vi "BuildMenu3.vi"(8 "Click Type":T1, 9 "Point":T2, 10 "XRef":refnum<vi>, 11 "State In":T10={"Input Type"=variant(dbl 0.0), "Width"=0, "Typedef Name"="", "Value Type"=variant, "Selection"=0, "Options"=[], "Selections"=[], "Display Selections"=[], "Element Names"=[], "Typedef Name Width"=0, "Display Selection Width"=[], "Code Generated"=FALSE, "Write Lock"=FALSE, "Is DVR"=FALSE}) -> (1 "Show Standard Items? (Popup click only)":bool=TRUE, 2 "Menu Specification":T4)   [LabVIEW 2015, in "Read-Write-Signals.xnode"]
doc: "This ability VI is used to describe the menu LabVIEW will display in response to a popup (right) click or a ShowMenu reply from OperateClick.\n \n Click Type is the type of click that led to this call of the ability. Point is the location of the user's popup click, and is relative to the top-left corner of your XNode's bounds. You may use this point to make your popup sensitive to the location that was clicked. Show Standard Items? is applicable only if Click Type is Popup, and tells LabVIEW whether it should include the standard popup items that are included on every node in LabVIEW.\n \n Menu Specification is an array of clusters describing the menu.\n Item: A string that will appear in the menu.\n Id: A string that identifies this item and will be passed to SelectMenu3.\n StartSub: The current string will be the header for a pull right menu.\n EndSub: The current string will be the last item in a pull right menu.\n Checked: The current item will have a check mark next to it.\n Disabled: The current item will be diabled and greyed out.\n Separator: The current item will be a separator. Item string is not displayed.\n Help: The text that should be displayed in context help when this menu item is hovered over. This functionality is currently not implemented.\n \n The index from this array will be an input to SelectMenu3.\n \n Remember to localize the strings in your menu.\n\nDefault behavior: Only show standard items for a popup click, show nothing for operate click.\n\nThis ability does not provide UI and OS messages are not handled.\n\nSee also: SelectMenu3"
uses:
  Read-Write-Signals.xnode
  State.ctl
  Read-Write-Signals Item.ctl
  Read-Write-Signals Sub Item.ctl
  Read-Write-Signals Sub Item Type.ctl
  Read-Write-Signals Selection.ctl
  Read-Write-Signals Display Selection.ctl
  <vilib>/XNodeSupport/XNodeMenuSpecs3.ctl
  <vilib>/XNodeSupport/XNodeMenuSpec3.ctl
  <vilib>/XNodeSupport/XNodeString.ctl
  <vilib>/XNodeSupport/XNodeBool.ctl
  <vilib>/XNodeSupport/XNodeStandardHelpInfo.ctl
  <vilib>/XNodeSupport/XNodePath.ctl
  <vilib>/XNodeSupport/XNodePoint.ctl
  <vilib>/XNodeSupport/XNodeInt.ctl
  <vilib>/XNodeSupport/XNodeClickTypes.ctl
  <vilib>/XNodeSupport/NI_XNodeSupport.lvlib
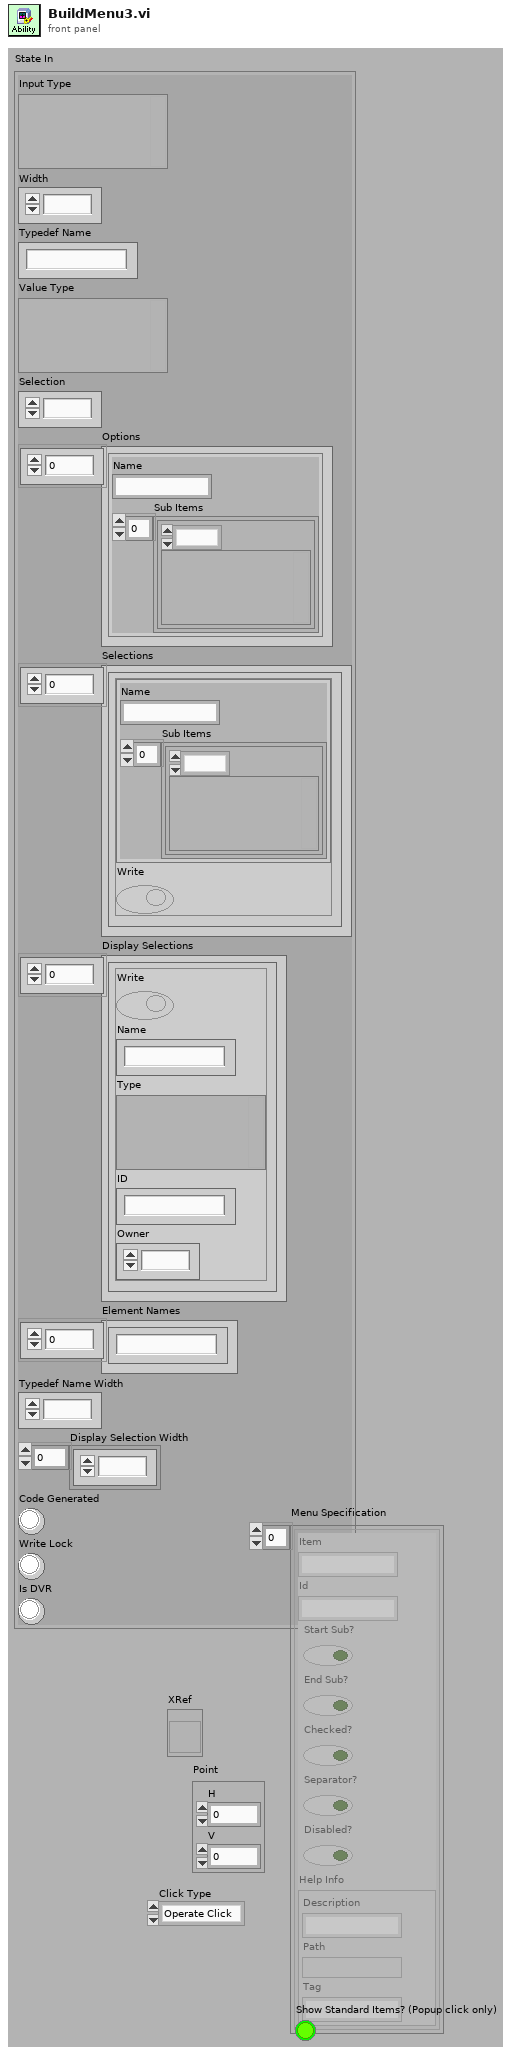
[diagram p1: front panel]
types:
  T1 = typedef "NI_XNodeSupport.lvlib/XNodeClickTypes.ctl" = enum32{"Operate Click", "Popup Click"}
  T2 = typedef "NI_XNodeSupport.lvlib/XNodePoint.ctl" = cluster{"H":T3, "V":T3}
  T3 = typedef "NI_XNodeSupport.lvlib/XNodeInt.ctl" = i32
  T4 = typedef "NI_XNodeSupport.lvlib/XNodeMenuSpecs3.ctl" = T5[]
  T5 = typedef "NI_XNodeSupport.lvlib/XNodeMenuSpec3.ctl" = cluster{"Item":T6, "Id":T6, "Start Sub?":T7, "End Sub?":T7, "Checked?":T7, "Separator?":T7, "Disabled?":T7, "Help Info":T8}
  T6 = typedef "NI_XNodeSupport.lvlib/XNodeString.ctl" = string
  T7 = typedef "NI_XNodeSupport.lvlib/XNodeBool.ctl" = bool
  T8 = typedef "NI_XNodeSupport.lvlib/XNodeStandardHelpInfo.ctl" = cluster{"Description":T6, "Path":T9, "Tag":T6}
  T9 = typedef "NI_XNodeSupport.lvlib/XNodePath.ctl" = path
  T10 = typedef "Read-Write-Signals.xnode/State.ctl" = cluster{"Input Type":variant, "Width":i32, "Typedef Name":string, "Value Type":variant, "Selection":i32, "Options":T11[], "Selections":T14[], "Display Selections":T15[], "Element Names":string[], "Typedef Name Width":i32, "Display Selection Width":i32[], "Code Generated":bool, "Write Lock":bool, "Is DVR":bool}
  T11 = typedef "Read-Write-Signals Item.ctl" = cluster{"Name":string, "Sub Items":T12[]}
  T12 = typedef "Read-Write-Signals Sub Item.ctl" = cluster{"Type":T13, "Value":variant}
  T13 = typedef "Read-Write-Signals Sub Item Type.ctl" = enum8{"Cluster Element", "Array Element", "Subarray"}
  T14 = typedef "Read-Write-Signals Selection.ctl" = cluster{"Item":T11, "Write":bool}
  T15 = typedef "Read-Write-Signals Display Selection.ctl" = cluster{"Write":bool, "Name":string, "Type":variant, "ID":string, "Owner":i32}
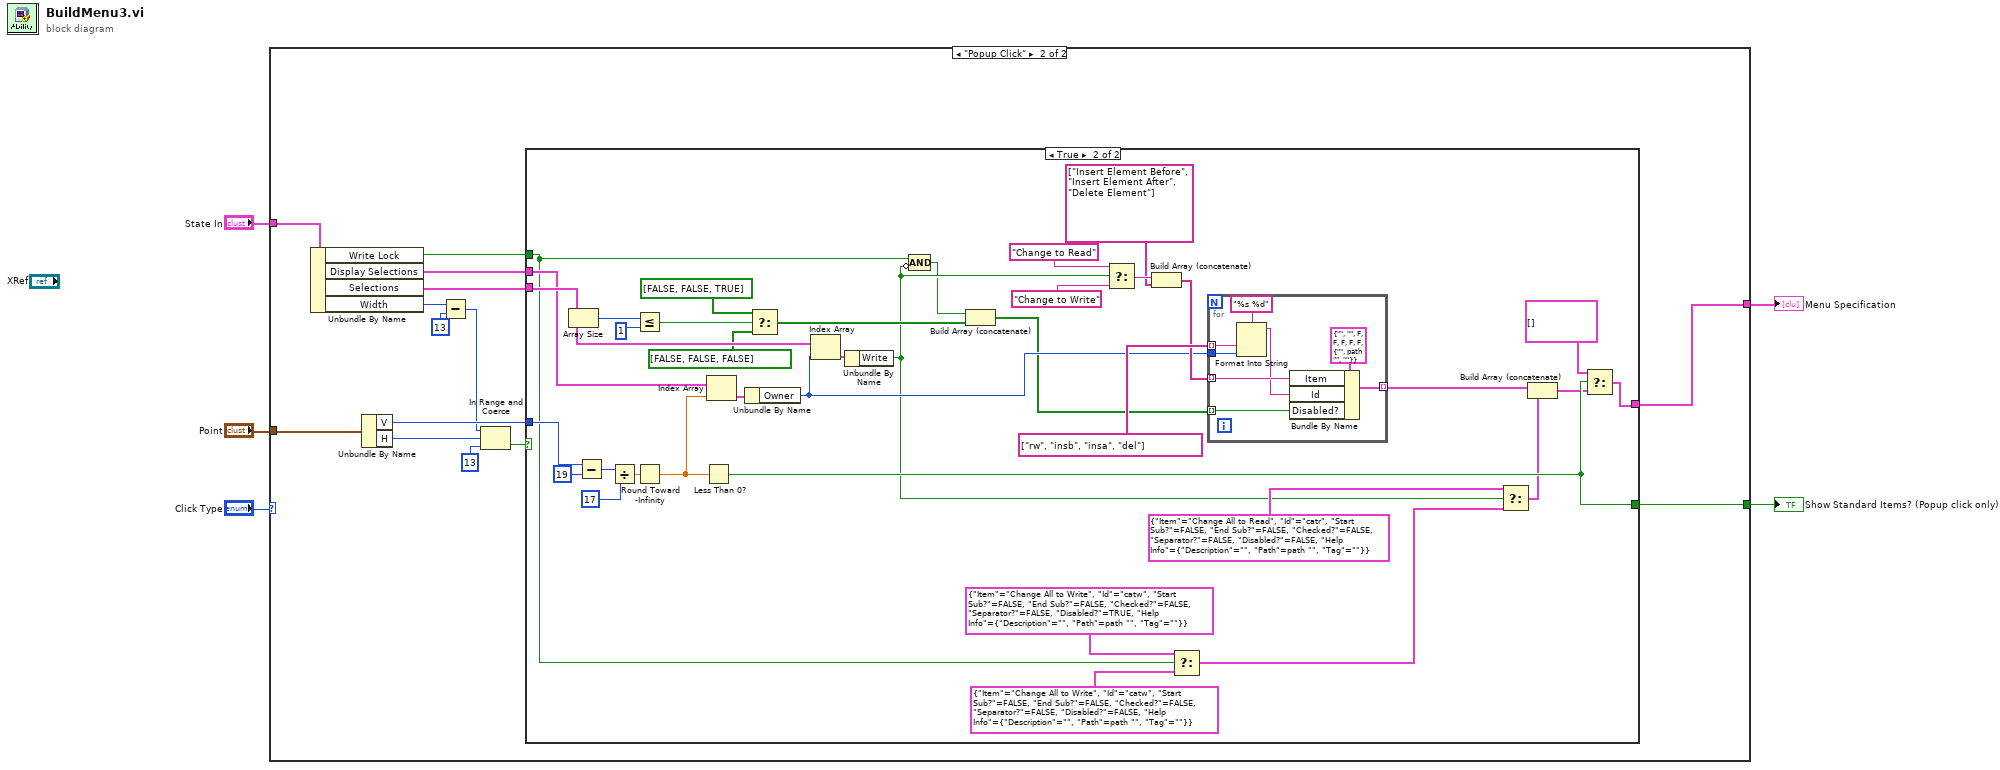
[diagram p0: block diagram]
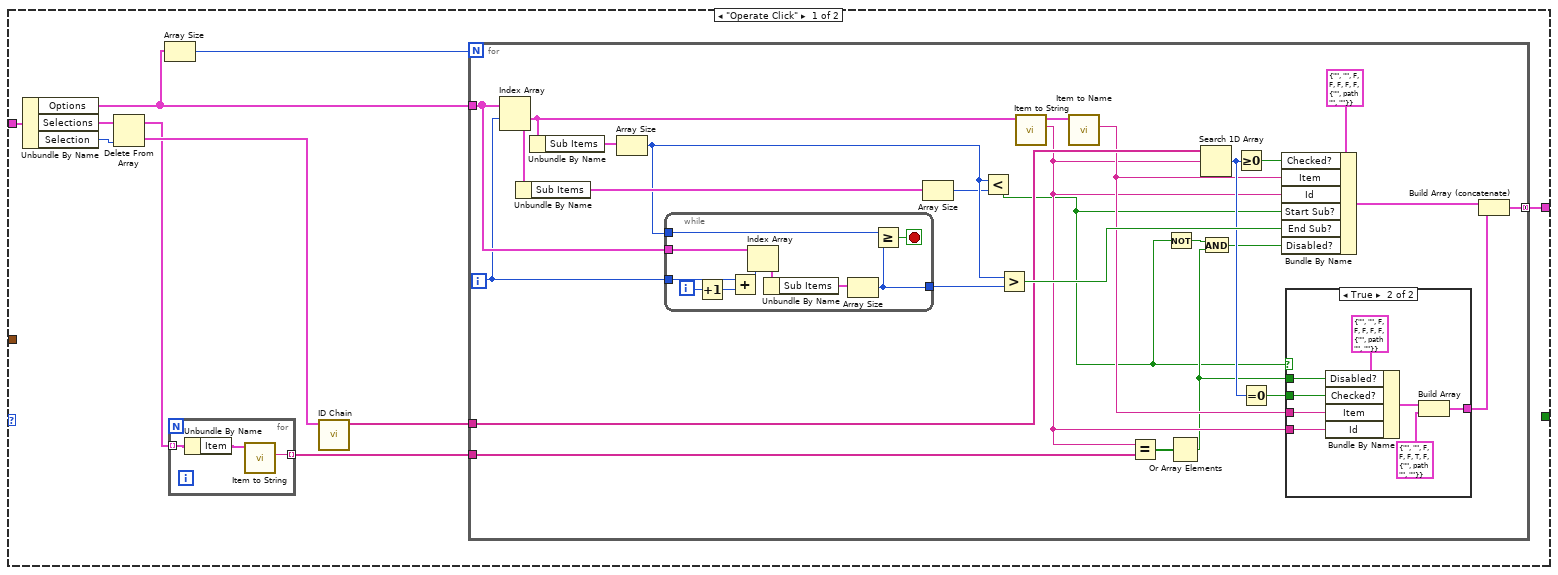
[diagram p2: hidden frame]
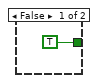
[diagram p4: hidden frame]
diagram:
  n1 = case shown="\"Popup Click\"" "Click Type" {
    tunnel: "State In" -> [w15 w76]
    tunnel: [w6 w72] -> w2
    tunnel: "Point" -> [_ w75]
    tunnel: [_ w73] -> w1
    frame "Operate Click" {
      n2 = Unbundle By Name(w15) -> ("Options"=w13:T11[], "Selections"=w10:T14[], "Selection"=w9:i32)
      n3 = Delete From Array(array=w10, index=w9) -> (deleted portion=w11:T14, array with subset deleted=w8:T14[])  [unwired: 1 in]
      n4 = Array Size(array=w13) -> (size(s)=w14:i32)
      n5 = for {
        tunnel: w8 -> [w18] mode=indexing
        tunnel: [w16] -> w7 mode=indexing
        n6 = Unbundle By Name(w18) -> ("Item"=w17:T11)
        n7 = call "Item to String.vi"("Item in"=w17) -> ("0 String"=w16:string)  [unwired: 9 in, 1 out]
      }
      n8 = call "ID Chain.vi"("Selection"=w11) -> ("Array"=w12:string[])  [unwired: 10 in]
      n9 = for {
        N: w14 -> [_]
        tunnel: w13 -> [w23]
        tunnel: [w37] -> w6 mode=concatenating
        tunnel: w12 -> [w35]
        tunnel: w7 -> [w31]
        i -> [w22]
        n10 = Index Array(array=w23, index #1=w22) -> (element #1=w43:T11, element #2=w42:T11)  [unwired: 1 in]
        n11 = Unbundle By Name(w42) -> ("Sub Items"=w36:T12[])
        n12 = Unbundle By Name(w43) -> ("Sub Items"=w41:T12[])
        n13 = Array Size(array=w41) -> (size(s)=w21:i32)
        n14 = while {
          tunnel: w23 -> [w55]
          tunnel: w22 -> [w54]
          tunnel: w21 -> [w46]
          tunnel: [w47] -> w19
          i -> [w53]
          stop <- w48 stop-if-true
          n15 = Increment(x=w53) -> (x+1=w52:i32)
          n16 = Add(x=w54, y=w52) -> (x+y=w51:i32)
          n17 = Index Array(array=w55, index=w51) -> (element=w49:T11)
          n18 = Unbundle By Name(w49) -> ("Sub Items"=w50:T12[])
          n19 = Array Size(array=w50) -> (size(s)=w47:i32)
          n20 = Greater Or Equal?(x=w46, y=w47) -> (x >= y?=w48:bool)
        }
        n21 = Array Size(array=w36) -> (size(s)=w20:i32)
        n22 = Less?(x=w21, y=w20) -> (x < y?=w24:bool)
        n23 = Greater?(x=w21, y=w19) -> (0:w40:bool)
        n24 = call "Item to String.vi"("Item in"=w43) -> ("0 String"=w28:string, "Item out"=w45:T11)  [unwired: 9 in]
        n25 = call "Item to Name.vi"("Item in"=w45) -> ("Display Name"=w30:string)  [unwired: 9 in, 1 out]
        n26 = Equal?(x=w28, y=w31) -> (x = y?=w29:bool[])
        n27 = Not(x=w24) -> (.not. x?=w25:bool)
        n28 = Or Array Elements(Boolean array=w29) -> (logical OR=w27:bool)
        n29 = Search 1D Array(1D array=w35, element=w28) -> (index of element=w32:i32)  [unwired: 1 in]
        n30 = And(x=w25, y=w27) -> (x .and. y?=w26:bool)
        n31 = Greater Or Equal To 0?(x=w32) -> (x >= 0?=w34:bool)
        n32 = Equal To 0?(x=w32) -> (x = 0?=w33:bool)
        n33 = Bundle By Name(cluster=T5 {"Item"="", "Id"="", "Start Sub?"=FALSE, "End Sub?"=FALSE, "Checked?"=FALSE, "Separator?"=FALSE, "Disabled?"=FALSE, "Help Info"={"Description"="", "Path"=path "", "Tag"=""}} ("Menu Item 3"), "Checked?"=w34, "Item"=w30, "Id"=w28, "Start Sub?"=w24, "End Sub?"=w40, "Disabled?"=w26) -> (w38:T5)
        n34 = case shown="True" w24 {
          tunnel: w30 -> [_ w63]
          tunnel: w28 -> [_ w62]
          tunnel: [_ w58] -> w39
          tunnel: w33 -> [_ w57]
          tunnel: w27 -> [_ w56]
          frame False {
          }
          frame True {
            n35 = Bundle By Name(cluster=T5 {"Item"="", "Id"="", "Start Sub?"=FALSE, "End Sub?"=FALSE, "Checked?"=FALSE, "Separator?"=FALSE, "Disabled?"=FALSE, "Help Info"={"Description"="", "Path"=path "", "Tag"=""}} ("Menu Item 3"), "Disabled?"=w56, "Checked?"=w57, "Item"=w63, "Id"=w62) -> (w61:T5)
            n36 = Build Array(w61, T5 {"Item"="", "Id"="", "Start Sub?"=FALSE, "End Sub?"=FALSE, "Checked?"=FALSE, "Separator?"=TRUE, "Disabled?"=FALSE, "Help Info"={"Description"="", "Path"=path "", "Tag"=""}} ("Menu Item 3")) -> (w58:T5[])
          }
        }
        n37 = Build Array (concatenate)(w38, w39) -> (w37:T5[])
      }
    }
    frame "Popup Click" {
      n38 = Unbundle By Name(w76) -> ("Write Lock"=w64:bool, "Display Selections"=w65:T15[], "Selections"=w74:T14[], "Width"=w70:i32)
      n39 = Unbundle By Name(w75) -> ("V"=w77:T3, "H"=w71:T3)
      n40 = Subtract(x=w70, y=13) -> (x-y=w68:i32)
      n41 = In Range and Coerce(upper limit=w68, x=w71, lower limit=T3 13) -> (In Range?=w66:bool)  [unwired: 1 out]
      n42 = case shown="True" w66 {
        tunnel: w77 -> [_ w112]
        tunnel: w74 -> [_ w97]
        tunnel: [TRUE w108] -> w73
        tunnel: [_ w103] -> w72
        tunnel: w65 -> [_ w90]
        tunnel: w64 -> [_ w82]
        frame False {
        }
        frame True {
          n43 = Array Size(array=w97) -> (size(s)=w96:i32)
          n44 = Subtract(x=w112, y=T3 19) -> (x-y=w115:T3)
          n45 = Divide(x=w115, y=T3 17) -> (x/y=w113:dbl)
          n46 = Less Or Equal?(x=w96, y=1 ("x")) -> (x <= y?=w94:bool)
          n47 = Round Toward -Infinity(1:w113) -> (0:w109:dbl)
          n48 = Less Than 0?(x=w109) -> (x < 0?=w108:bool)
          n49 = Index Array(array=w90, index=w109) -> (element=w110:T15)
          n50 = Unbundle By Name(w110) -> ("Owner"=w86:i32)
          n51 = Select(t=bool[] [FALSE, FALSE, TRUE], s=w94, f=bool[] [FALSE, FALSE, FALSE]) -> (s? t:f=w91:bool[])
          n52 = Index Array(array=w97, index=w86) -> (element=w107:T14)
          n53 = Unbundle By Name(w107) -> ("Write"=w81:bool)
          n54 = Compound Arithmetic op=AND(w82, invert w81) -> (w79:bool)
          n55 = Build Array (concatenate)(w79, w91) -> (w80:bool[])
          n56 = Select(t=T6 "Change to Read" ("Item"), s=w81, f=T6 "Change to Write" ("Item")) -> (s? t:f=w100:T6)
          n57 = Build Array (concatenate)(w100, string[] ["Insert Element Before", "Insert Element After", "Delete Element"]) -> (w98:T6[])
          n58 = Select(t=T5 {"Item"="Change All to Write", "Id"="catw", "Start Sub?"=FALSE, "End Sub?"=FALSE, "Checked?"=FALSE, "Separator?"=FALSE, "Disabled?"=TRUE, "Help Info"={"Description"="", "Path"=path "", "Tag"=""}} ("Menu Item 3"), s=w82, f=T5 {"Item"="Change All to Write", "Id"="catw", "Start Sub?"=FALSE, "End Sub?"=FALSE, "Checked?"=FALSE, "Separator?"=FALSE, "Disabled?"=FALSE, "Help Info"={"Description"="", "Path"=path "", "Tag"=""}} ("Menu Item 3")) -> (s? t:f=w83:T5)
          n59 = for {
            tunnel: w86 -> [w122]
            tunnel: string[] ["rw", "insb", "insa", "del"] -> [w121] mode=indexing
            tunnel: [w119] -> w101 mode=indexing
            tunnel: w98 -> [w118] mode=indexing
            tunnel: w80 -> [w116] mode=indexing
            n60 = Format Into String(format string="%s %d", w121, w122) -> (resulting string=w117:string)  [unwired: 2 in, 1 out]
            n61 = Bundle By Name(cluster=T5 {"Item"="", "Id"="", "Start Sub?"=FALSE, "End Sub?"=FALSE, "Checked?"=FALSE, "Separator?"=FALSE, "Disabled?"=FALSE, "Help Info"={"Description"="", "Path"=path "", "Tag"=""}} ("Menu Item 3"), "Item"=w118, "Id"=w117, "Disabled?"=w116) -> (w119:T5)
          }
          n62 = Select(t=T5 {"Item"="Change All to Read", "Id"="catr", "Start Sub?"=FALSE, "End Sub?"=FALSE, "Checked?"=FALSE, "Separator?"=FALSE, "Disabled?"=FALSE, "Help Info"={"Description"="", "Path"=path "", "Tag"=""}} ("Menu Item 3"), s=w81, f=w83) -> (s? t:f=w88:T5)
          n63 = Build Array (concatenate)(w101, w88) -> (w89:T5[])
          n64 = Select(t=T4 [], s=w108, f=w89) -> (s? t:f=w103:T4)
        }
      }
    }
  }
  "Menu Specification" <- w2
  "Show Standard Items? (Popup click only)" <- w1
